vi "Set focus speed.vi"(8 "error in (no error)":errorcluster, 11 "ImageStack in":refnum<class "ImageStack.lvclass">) -> (0 "error out":errorcluster, 3 "ImageStack out":refnum<class "ImageStack.lvclass">)   [LabVIEW 2012, in "ImageStack.lvclass"]
uses:
  ImageStack.lvclass
  ImageStack.lvclass/ImageStack.ctl
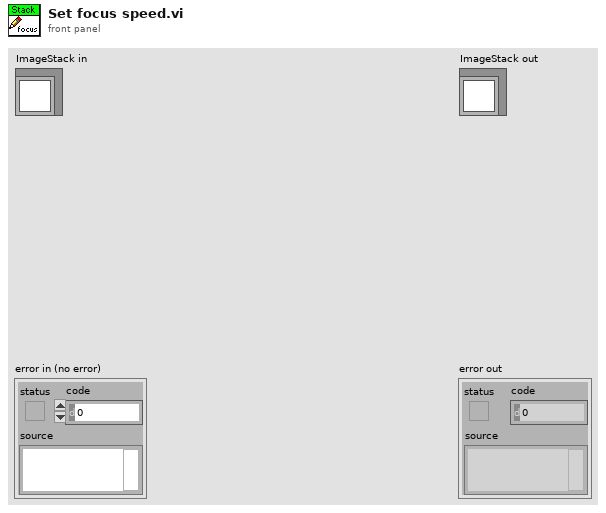
[diagram p1: front panel]
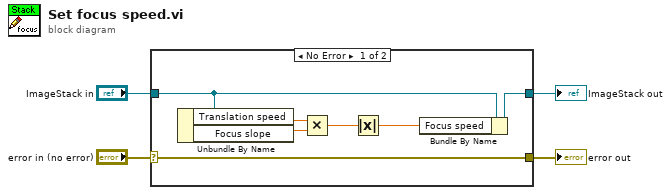
[diagram p0: block diagram]
diagram:
  n1 = case shown="No Error" "error in (no error)" {
    selector: "error in (no error)" -> [w11 w13]
    tunnel: [w11 w13] -> w3
    tunnel: [w9 w12] -> w1
    tunnel: "ImageStack in" -> [w10 w12]
    frame No Error {
      n2 = Unbundle By Name(w10) -> ("Translation speed"=w8:dbl[unit], "Focus slope"=w7:dbl)
      n3 = Multiply(x=w8, y=w7) -> (x*y=w6:dbl[unit])
      n4 = Absolute Value(x=w6) -> (abs(x)=w5:dbl[unit])
      n5 = Bundle By Name(cluster=w10, "Focus speed"=w5) -> (w9:refnum<class "ImageStack.lvclass">)
    }
    frame Error {
    }
  }
  "error out" <- w3
  "ImageStack out" <- w1
